vi "AssertVIFPStateInvalid.vi"(0 "VI Reference In":refnum<vi>, 1 "Label":string, 3 "Assert Only? (F)":bool, 11 "Error In":errorcluster, 12 "Assert Interval(10 ms)":u32=10, 13 "Timeout(5 sec)":dbl=5.0) -> (4 "VI Reference Out":refnum<vi>, 6 "Asserted Value":T1(ring), 15 "Error Out":errorcluster)   [LabVIEW 2016, in "Drona.lvlib" / "AssertVI.lvlib"]
doc: "Asserts if the Front panel of the VI is in Invalid state.\nThe input control name is given as a string , incase of path, use delimiters inbetween the path."
uses:
  AssertVI.lvlib
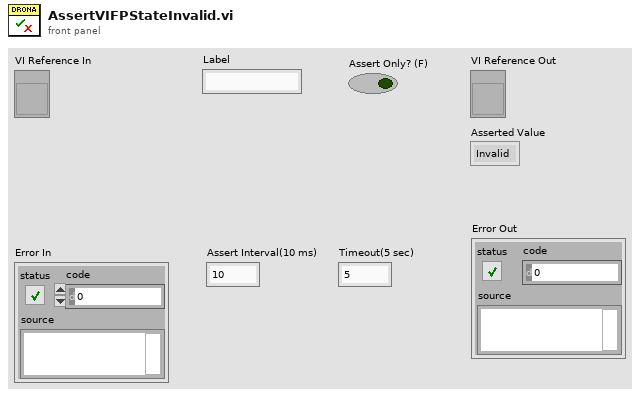
[diagram p1: front panel]
types:
  T1 = enum32{"Invalid", "Standard", "Closed", "Hidden", "Minimized", "Maximized"}
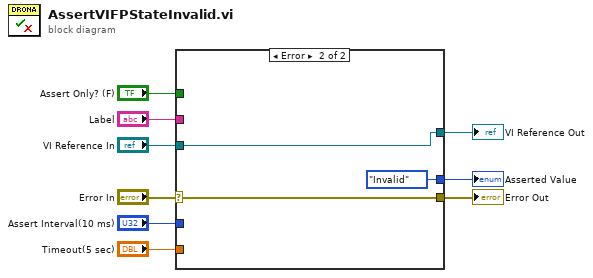
[diagram p0: block diagram]
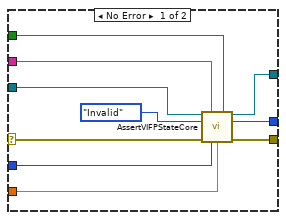
[diagram p2: hidden frame]
diagram:
  n1 = case shown="Error" "Error In" {
    selector: "Error In" -> [w19 w22]
    tunnel: [w18 w22] -> w8
    tunnel: "VI Reference In" -> [w17 w21]
    tunnel: "Label" -> [w16 _]
    tunnel: "Assert Only? (F)" -> [w10 _]
    tunnel: "Assert Interval(10 ms)" -> [w15 _]
    tunnel: "Timeout(5 sec)" -> [w14 _]
    tunnel: [w13 w21] -> w2
    tunnel: [w11 T1."Invalid" ("Asserted Value")] -> w1
    frame No Error {
      n2 = call "AssertVIFPStateCore.vi"("VI Reference In"=w17, "Label"=w16, "Assert Only? (F)"=w10, "FP State"=T1."Invalid", "Error In"=w19, "Assert Interval(10 ms)"=w15, "Timeout(5 sec)"=w14) -> ("VI Reference Out"=w13:refnum<vi>, "Asserted Value"=w11:T1, "Error Out"=w18:errorcluster)  [unwired: 6 in]
    }
    frame Error {
    }
  }
  "Error Out" <- w8
  "VI Reference Out" <- w2
  "Asserted Value" <- w1
